vi "TCL Get Current Signal.vi"(2 "error in (no error)":errorcluster, 3 "signal name":string, 4 "event number":i32) -> (0 "error out":errorcluster, 1 "signal":dbl[](array[numeric]))   [LabVIEW 2010]
uses:
  TCL Global.vi
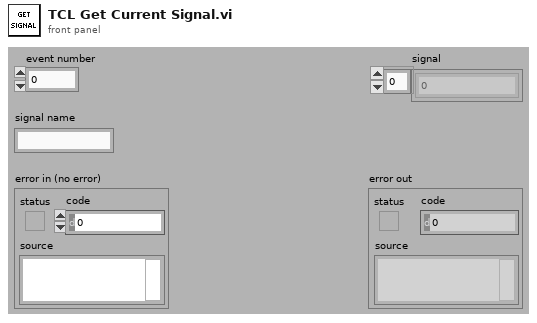
[diagram p1: front panel]
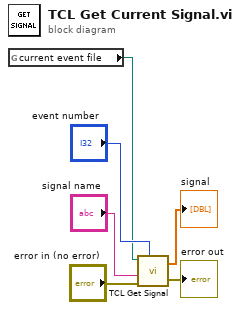
[diagram p0: block diagram]
diagram:
  n1 = global read "TCL Global.vi" "current event file"() -> (w5:path)
  n2 = call "TCL Get Signal.vi"("event number"="event number", "error in (no error)"="error in (no error)", "signal name"="signal name", "event file"=w5) -> ("error out"=→"error out":errorcluster, "signal"=→"signal":dbl[])  [unwired: 2 in]
